vi "CamTempTest2013.vi"() -> ()   [LabVIEW 2013]
panel:
  out "Total Nuber of Devices or DLLs":u32
  out "Device ID from \"GetIDs\"":u32
  out "Camera Handle":u32
  out "Versions":T1
  out "Device from ToolkitVersions":u32
  in  "Index":u32
  in  "Camera Index":u32=1 min=1 step=1
  in  "error in":errorcluster
  out "Number of Cameras":i32
  out "Toolkit Error":bool
  out "error out":errorcluster
  in  "stop":bool
  out "Waveform Chart":dbl(graph)
  out "Temperature":dbl
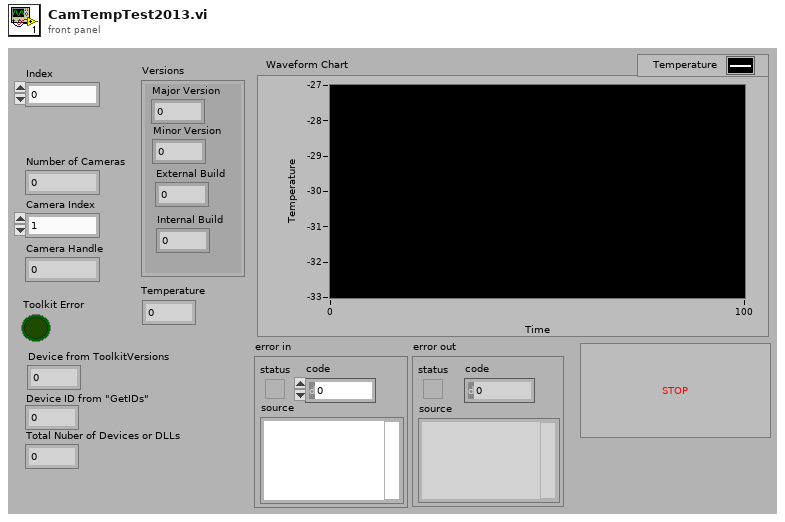
[diagram p1: front panel]
types:
  T1 = cluster{"Major Version":u32, "Minor Version":u32, "External Build":u32, "Internal Build":u32}
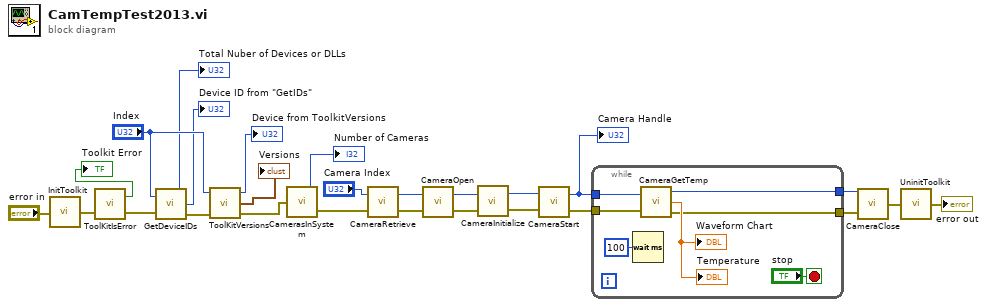
[diagram p0: block diagram]
diagram:
  n1 = call <userlib>:"InitToolkit.vi"("error in"="error in") -> ("error out"=w22:errorcluster)
  n2 = call <userlib>:"ToolKitIsError.vi"("error in"=w22) -> ("error out"=w12:errorcluster, "Error Flag"=→"Toolkit Error":bool)  [unwired: 1 in]
  n3 = call <userlib>:"GetDeviceIDs.vi"("Index"="Index", "error in"=w12) -> ("Total Nuber of Devices or DLLs"=→"Total Nuber of Devices or DLLs":u32, "Device ID"=→"Device ID from \"GetIDs\"":u32, "error out"=w11:errorcluster)
  n4 = call <userlib>:"ToolKitVersions.vi"("error in"=w11, "Index"="Index") -> ("error out"=w10:errorcluster, "Versions"=→"Versions":T1, "Device"=→"Device from ToolkitVersions":u32)  [unwired: 1 in]
  n5 = call <userlib>:"CamerasInSystem.vi"("error in"=w10) -> ("Number of Cameras"=→"Number of Cameras":i32, "error out"=w15:errorcluster)
  n6 = call <userlib>:"CameraRetrieve.vi"("error in"=w15, "Camera Index"="Camera Index") -> ("error out"=w21:errorcluster, "Device ID"=w20:u32)
  n7 = call <userlib>:"CameraOpen.vi"("error in"=w21, "Camera Device ID"=w20) -> ("error out"=w19:errorcluster, "Camera Handle"=w18:u32)
  n8 = call <userlib>:"CameraInitialize.vi"("error in"=w19, "Camera Handle"=w18) -> ("error out"=w17:errorcluster, "Camera Handle"=w16:u32)
  n9 = call <userlib>:"CameraStart.vi"("error in"=w17, "Camera Handle"=w16) -> ("error out"=w6:errorcluster, "Camera Handle"=w5:u32)
  "Camera Handle" <- w5
  n10 = while {
    tunnel: [w30] -> w24
    tunnel: [w29] -> w23
    tunnel: w5 -> [w28]
    tunnel: w6 -> [w27]
    stop <- "stop" stop-if-true
    n11 = Wait (ms)(milliseconds to wait=u32 100) -> ()  [unwired: 1 out]
    n12 = call <userlib>:"CameraGetTemp.vi"("Camera Handle"=w28, "error in (no error)"=w27) -> ("Camera Handle"=w30:u32, "Temperature"=→"Temperature" →"Waveform Chart":dbl, "error out"=w29:errorcluster)
  }
  n13 = call <userlib>:"CameraClose.vi"("error in"=w23, "Camera Handle"=w24) -> ("error out"=w26:errorcluster)
  n14 = call <userlib>:"UninitToolkit.vi"("error in"=w26) -> ("error out"=→"error out":errorcluster)
